vi "FTW-Listener-Construct.vi"(0 "FTW-Listener-TCP In":refnum<class "FTW-Listener-TCP.lvclass">, 5 "Address":string, 11 "error in":errorcluster) -> (4 "FTW-Listener-TCP Out":refnum<class "FTW-Listener-TCP.lvclass">, 15 "error out":errorcluster)   [LabVIEW 2013, in "FTW-Listener-TCP.lvclass"]
uses:
  FTW-Listener-TCP.lvclass
  Listener/FTW-Listener.lvclass
  FTW-Listener-TCP.lvclass/FTW-Listener-TCP.ctl
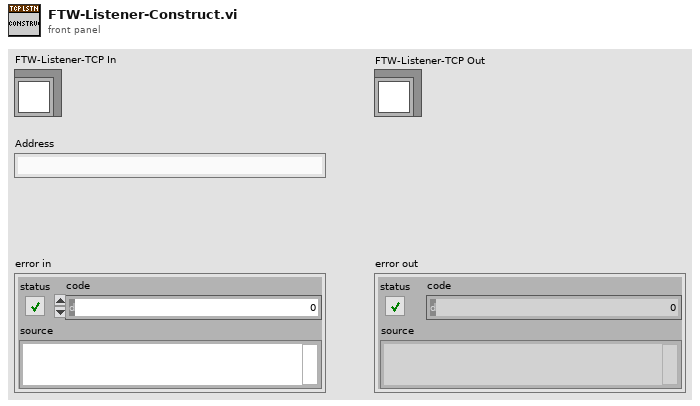
[diagram p1: front panel]
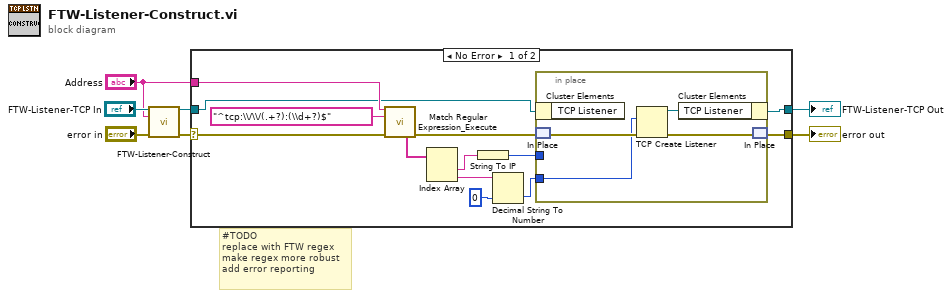
[diagram p0: block diagram]
diagram:
  # "#TODO\nreplace with FTW regex\nmake regex more robust\nadd error reporting"
  n1 = call-parent "FTW-Listener-Construct.vi"("Gmsg_Listener In"="FTW-Listener-TCP In", "Address"="Address", "error in"="error in") -> ("Gmsg_Listener Out"=w2:refnum<class "FTW-Listener-TCP.lvclass">, "error out"=w4:errorcluster)  [unwired: 11 in]
  n2 = case shown="No Error" w4 {
    selector: w4 -> [w16 w26]
    tunnel: [w20 w26] -> w6
    tunnel: [w19 w25] -> w5
    tunnel: "Address" -> [w17 _]
    tunnel: w2 -> [w8 w25]
    frame No Error {
      n3 = call <vilib>:"Match Regular Expression_Execute.vi"("input string"=w17, "regular expression"="^tcp:\\/\\/(.+?):(\\d+?)$" ("input string"), "error in (no error)"=w16) -> ("matched substrings"=w14:string[], "error out"=w15:errorcluster)  [unwired: 7 in, 4 out]
      n4 = Index Array(array=w14) -> (element #1=w13:string, element #2=w12:string)  [unwired: 2 in]
      n5 = String To IP(1:w13) -> (0:w9:u32)
      n6 = Decimal String To Number(string=w12, default (0L)=u16 0 ("remote port or service name")) -> (number=w10:u16)  [unwired: 1 in, 1 out]
      n7 = in-place {
        in-place-border: w9 -> [_]
        in-place-border: w10 -> [w21]
        n8 = in-place-cluster #1(w8) -> ()  [unwired: 1 out]
        n9 = in-place-match #2(w15) -> (w24:errorcluster)
        n10 = TCP Create Listener(8:w24, 10:w21) -> (0:w23:errorcluster, 3:w22:refnum<k5>)  [unwired: 3 in, 1 out]
        n11 = in-place-cluster #1("TCP Listener"=w22) -> (w19:refnum<class "FTW-Listener-TCP.lvclass">)
        n12 = in-place-match #2(w23) -> (w20:errorcluster)
      }
    }
    frame Error {
    }
  }
  "FTW-Listener-TCP Out" <- w5
  "error out" <- w6
